vi "_Get UserEvent.vi"(8 "error in (no error)":errorcluster, 11 "Event in":refnum<class "Event.lvclass">) -> (0 "error out":errorcluster, 2 "UserEvent":refnum<user-event>, 3 "Event out":refnum<class "Event.lvclass">)   [LabVIEW 2021, in "EventManagerLibrary.lvlib" / "Event.lvclass"]
uses:
  Event.lvclass
  EventDataObject/EventData.lvclass
  Event.lvclass/Event.ctl
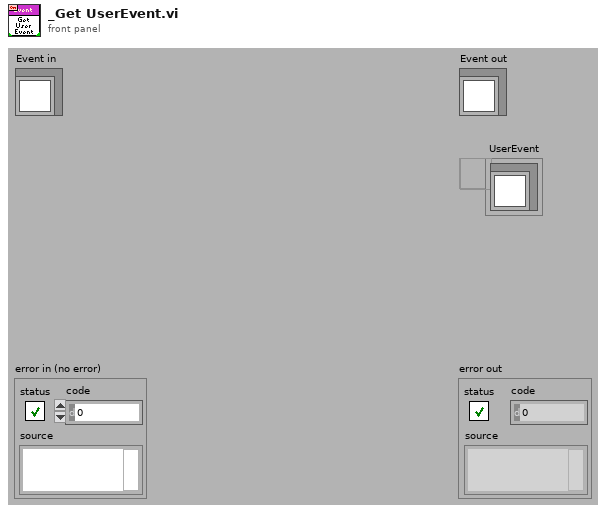
[diagram p1: front panel]
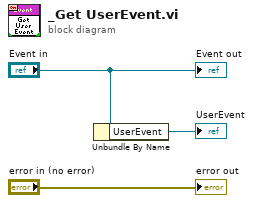
[diagram p0: block diagram]
diagram:
  n1 = Unbundle By Name("Event in") -> ("UserEvent"=→"UserEvent":refnum<user-event>)
  "error out" <- "error in (no error)"
  "Event out" <- "Event in"
